vi "VG_HYDRAU.vi"() -> ()   [LabVIEW 2020]
panel:
  out "CONTI HYDRAU":dbl
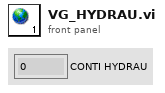
[diagram p1: front panel]
diagram:
